vi "Configure Delay Measurement.vi"(5 "Delay Measurement Type (0: Immediate)":i32(ring) items=["Immediate", "Normal"], 6 "Destination Waveform Direction (1: Forwards)":i32(ring)=1 items=["Backwards", "Forwards"], 7 "Measurement Number (0: Measurement 1)":i32(ring) items=["Measurement 1", "Measurement 2", "Measurement 3", "Measurement 4"], 8 "error in (no error)":errorcluster, 9 "Destination Waveform Slope (1: Rising)":i32(ring)=1 items=["Falling", "Rising"], 10 "Source Waveform Slope (1: Rising)":i32(ring)=1 items=["Falling", "Rising"], 11 "VISA resource name":refnum<visa-resource-name>) -> (0 "error out":errorcluster, 3 "VISA resource name out":refnum<visa-resource-name>)   [LabVIEW 2016, in "Tektronix DPO MSO 2000 4000 Series.lvlib"]
doc: "Configures the parameters for delay measurement or immediate delay measurement."
uses:
  Tektronix DPO MSO 2000 4000 Series.lvlib
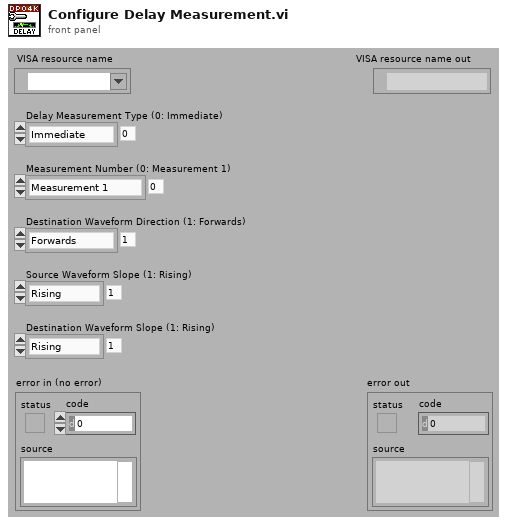
[diagram p1: front panel]
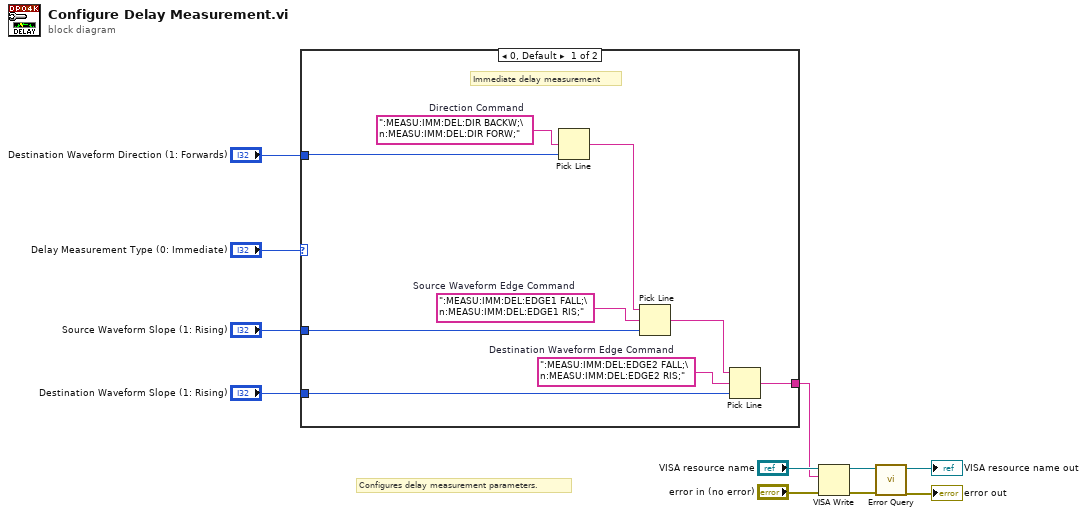
[diagram p0: block diagram]
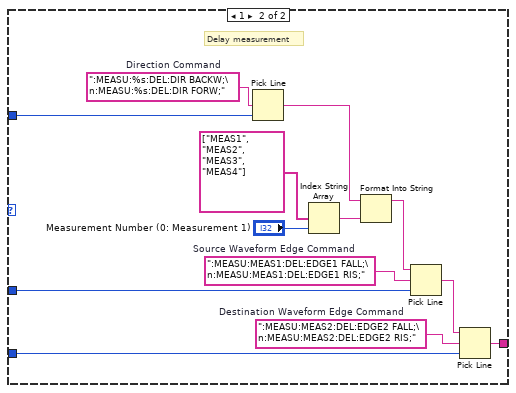
[diagram p2: hidden frame]
diagram:
  # "Configures delay measurement parameters."
  n1 = case shown="0, Default" "Delay Measurement Type (0: Immediate)" {
    tunnel: "Source Waveform Slope (1: Rising)" -> [w19 w30]
    tunnel: "Destination Waveform Slope (1: Rising)" -> [w17 w32]
    tunnel: "Destination Waveform Direction (1: Forwards)" -> [w15 w29]
    tunnel: [w12 w21] -> w1
    frame 0, Default {
      w16 = ":MEASU:IMM:DEL:DIR BACKW;\n:MEASU:IMM:DEL:DIR FORW;"  # Direction Command
      w18 = ":MEASU:IMM:DEL:EDGE2 FALL;\n:MEASU:IMM:DEL:EDGE2 RIS;"  # Destination Waveform Edge Command
      w20 = ":MEASU:IMM:DEL:EDGE1 FALL;\n:MEASU:IMM:DEL:EDGE1 RIS;"  # Source Waveform Edge Command
      # "Immediate delay measurement"
      n2 = Pick Line(multi-line string=w16, line index=w15) -> (output string=w14:string)  [unwired: 1 in]
      n3 = Pick Line(string ("")=w14, multi-line string=w20, line index=w19) -> (output string=w13:string)
      n4 = Pick Line(string ("")=w13, multi-line string=w18, line index=w17) -> (output string=w12:string)
    }
    frame 1 {
      w28 = ":MEASU:%s:DEL:DIR BACKW;\n:MEASU:%s:DEL:DIR FORW;"  # Direction Command
      w31 = ":MEASU:MEAS1:DEL:EDGE1 FALL;\n:MEASU:MEAS1:DEL:EDGE1 RIS;"  # Source Waveform Edge Command
      w33 = ":MEASU:MEAS2:DEL:EDGE2 FALL;\n:MEASU:MEAS2:DEL:EDGE2 RIS;"  # Destination Waveform Edge Command
      # "Delay measurement"
      n5 = Pick Line(multi-line string=w28, line index=w29) -> (output string=w27:string)  [unwired: 1 in]
      n6 = Index String Array(1:"Measurement Number (0: Measurement 1)", 2:string[] ["MEAS1", "MEAS2", "MEAS3", "MEAS4"] ("string array")) -> (0:w24:string)  [unwired: 1 in]
      n7 = Format Into String(format string=w27, w24) -> (resulting string=w23:string)  [unwired: 2 in, 1 out]
      n8 = Pick Line(string ("")=w23, multi-line string=w31, line index=w30) -> (output string=w22:string)
      n9 = Pick Line(string ("")=w22, multi-line string=w33, line index=w32) -> (output string=w21:string)
    }
  }
  n10 = VISA Write(VISA resource name="VISA resource name", write buffer=w1, error in (no error)="error in (no error)") -> (VISA resource name out=w9:refnum<visa-resource-name>, error out=w8:errorcluster)  [unwired: 1 out]
  n11 = call "Error Query.vi"("error in (no error)"=w8, "VISA resource name"=w9) -> ("error out"=→"error out":errorcluster, "VISA resource name out"=→"VISA resource name out":refnum<visa-resource-name>)  [unwired: 6 in, 2 out]
